vi "initialize_driver_session.vi"(4 "Supported instruments":string[](array[string]), 5 "Repeated Capabilities":T3(array[cluster]), 6 "Attributes":T1(array[cluster]) {"Access" items=["Read Only", "Write Only", "Read/Write"]; "Data Type" items=["ViInt32", "ViReal64", "ViString", "ViBoolean", "None"]}, 7 "Range Tables":T2(array[cluster]) {"Type" items=["Range", "Coerced", "Discrete"]}, 8 "error in":errorcluster, 9 "Option String":string, 11 "VISA resource name":refnum<visa-resource-name>) -> (0 "error out":errorcluster, 2 "Simulation *IDN? response":string, 3 "VISA resource name out":refnum<visa-resource-name>)   [LabVIEW 2014, in "rszvl_rsidr_core.lvlib"]
uses:
  rszvl_rsidr_core.lvlib
  type_Session_Data.ctl
  type_Error_Codes.ctl
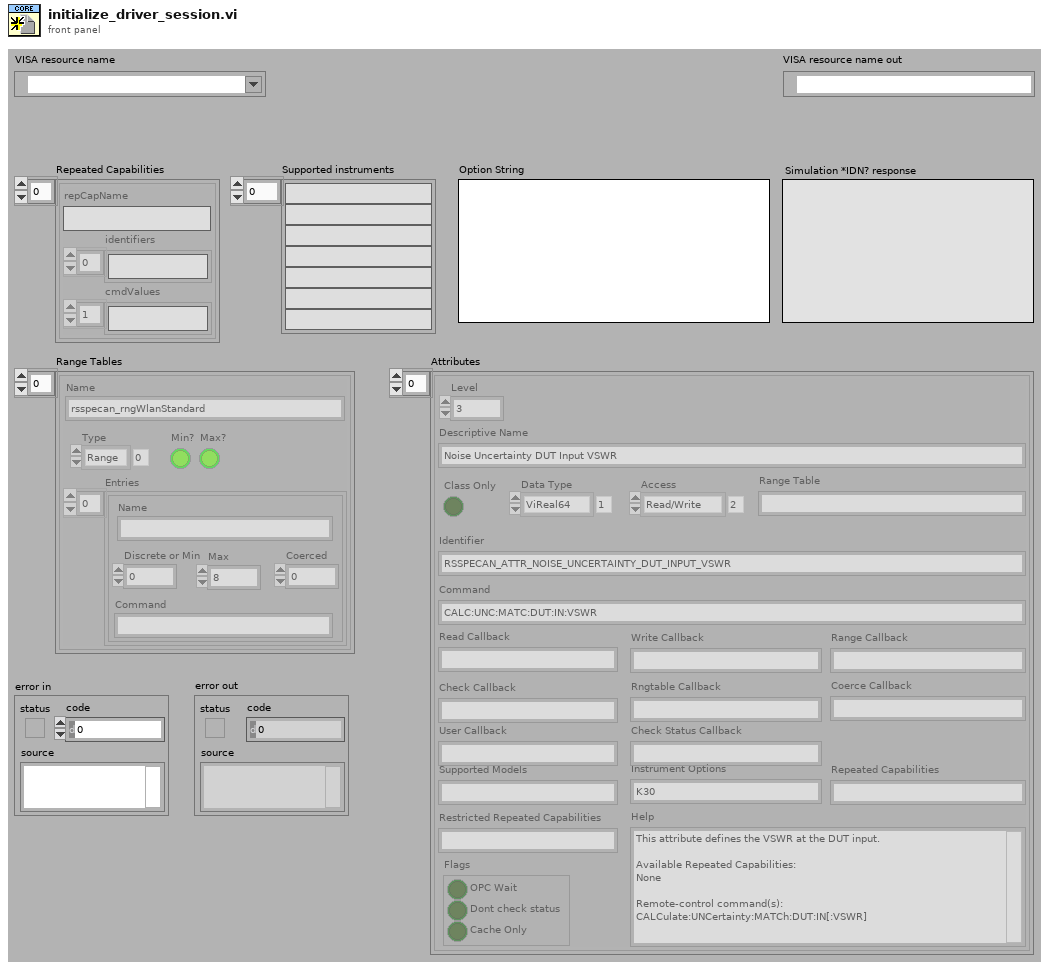
[diagram p1: front panel]
types:
  T1 = cluster{"Level":i32, "Descriptive Name":string, "Class Only":bool, "Data Type":u16, "Access":u16, "Identifier":string, "Range Table":string, "Command":string, "Read Callback":string, "Write Callback":string, "Range Callback":string, "Check Callback":string, "Rngtable Callback":string, "Coerce Callback":string, "User Callback":string, "Supported Models":string, "Instrument Options":string, "Repeated Capabilities":string, "Restricted Repeated Capabilities":string, "Help":string, "Flags":cluster{"OPC Wait":bool, "Dont check status":bool, "Cache Only":bool}, "Check Status Callback":string}[]
  T2 = cluster{"Name":string, "Type":i32, "Min?":bool, "Max?":bool, "Entries":cluster{"Name":string, "Discrete or Min":dbl, "Max":dbl, "Coerced":dbl, "Command":string}[]}[]
  T3 = cluster{"repCapName":string, "identifiers":string[], "cmdValues":string[]}[]
  T4 = typedef "rszvl_rsidr_core.lvlib/type_Error_Codes.ctl" = enum16{"No_error", "VISA_err_ResourceNotFound", "VISA_err_Timeout", "VISA_warn_MoreDataAvailable", "RS_err_MissingCallback", "RS_err_InvalidAttribute", "RS_err_InvalidValue", "RS_err_UnknownResource", "RS_err_AlreadyInitialized", "RS_err_InstrumentStatus", "RS_err_BadRepCapName", "RS_err_TypesMismatch", "RS_err_ValueNotSupported", "RS_err_InvalidRngTable", "RS_err_IDqueryFail", "RS_err_UnexpResponse", "VISA_warn_ConfigNotLoaded", "RS_err_AttributeNotReadable", "RS_err_AttributeNotWritable", "RS_err_InstrumentType", "RS_err_InstrumentOption", "VISA_err_InvalidSize", "RS_err_ReliabilityIndicator", "VISA_warn_UnknownStatus", "VISA_warn_TermCharRead", "VISA_err_IO_error"}
  T5 = enum16{"Initialize", "Check", "Get Numeric Value", "Get Default Value"}
  T6 = typedef "rszvl_rsidr_core.lvlib/type_Session_Data.ctl" = cluster{"Instr type":string, "Instr type for err. msg.":string, "Installed Options":string[], "OPC Timeout":i32, "Query Instrument Status":bool, "Check Range":bool, "Check Options":bool, "Add LF to Write":bool, "Simulate":bool, "Logging":bool, "Logging params":variant, "Interface Type":enum16{"Unknown", "GPIB", "VXI", "GPIB_VXI", "ASRL", "PXI", "TCPIP", "USB", "SOCKET"}, "Fast Sweep":i32, "AdditionalFlags":i32, "WaitBeforeWrite":i32, "WaitBeforeRead":i32, "BinDataChunkSize":i64}
  T7 = enum16{"Initialize", "GetData", "SetData", "Clear"}
  T8 = enum16{"Initialize", "Get Cached Value", "Set Cached Value", "Clear"}
  T9 = enum16{"Unknown", "GPIB", "VXI", "GPIB_VXI", "ASRL", "PXI", "TCPIP", "USB", "SOCKET"}
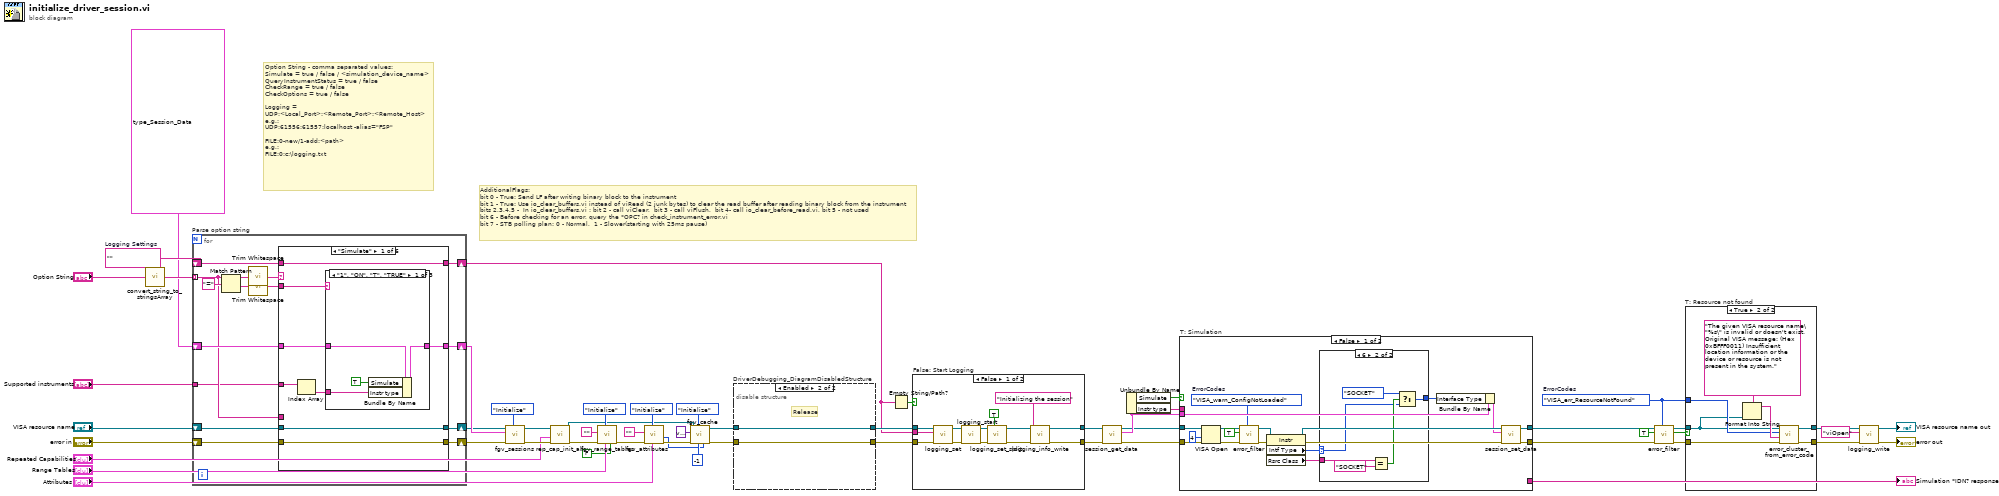
[diagram p0: block diagram]
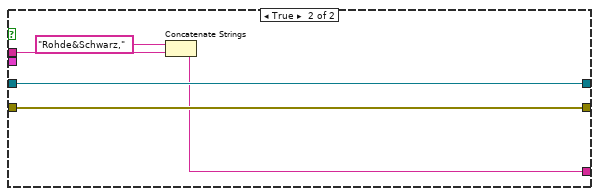
[diagram p3: hidden frame]
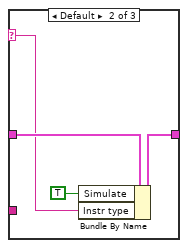
[diagram p6: hidden frame]
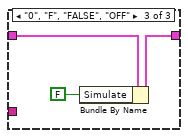
[diagram p7: hidden frame]
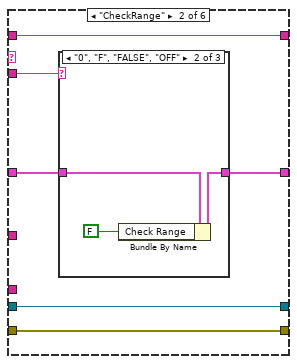
[diagram p8: hidden frame]
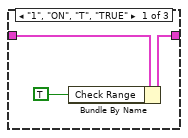
[diagram p9: hidden frame]
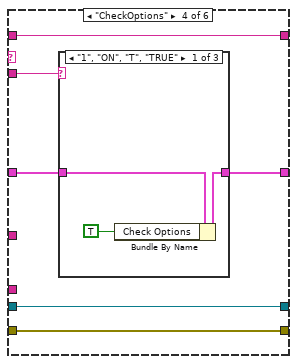
[diagram p12: hidden frame]
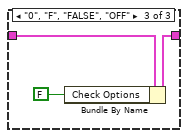
[diagram p14: hidden frame]
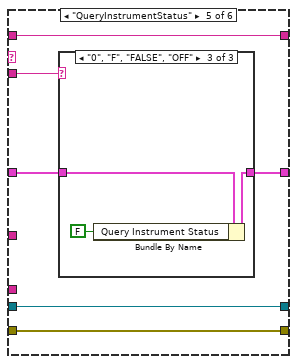
[diagram p15: hidden frame]
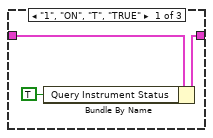
[diagram p16: hidden frame]
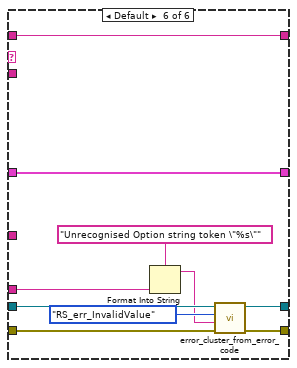
[diagram p18: hidden frame]
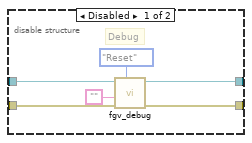
[diagram p19: hidden frame]
diagram:
  w17 = type_Error_Codes."VISA_err_ResourceNotFound"  # ErrorCodes
  w29 = ""  # Logging Settings
  # "AdditionalFlags:\nbit 0 - True: Send LF after writing binary block to the instrument\nbit 1 - True: Use io_clear_buffers.vi instead of viRead (2 junk bytes) to clear the read buffer after reading binary block from the instrument\nbits 2,3,4,5 -  In io_clear_buffers.vi : bit 2 - call viClear,  bit 3 - call viFlush,  bit 4- call io_clear_before_read.vi, bit 5 - not used\nbit 6 - Before checking for an error, query the *OPC? in check_instrument_error.vi\nbit 7 - STB polling plan: 0 - Normal,  1 - Slower(starting with 25ms pause)"
  # "Option String - comma separated values:\nSimulate = true / false / <simulation_device_name>\nQueryInstrumentStatus = true / false\nCheckRange = true / false\nCheckOptions = true / false\n\nLogging =\nUDP:<Local_Port>:<Remote_Port>:<Remote_Host>\ne.g.:\nUDP:61556:61557:localhost -alias=\"FSP\"\n\nFILE:0-new/1-add:<path>\ne.g.:\nFILE:0:c:\\logging.txt"
  n1 = call "convert_string_to_stringsArray.vi"("String in"="Option String") -> ("string array out"=w38:string[])  [unwired: 3 in, 1 out]
  n2 = for "Parse option string" {
    tunnel: w38 -> [w60] mode=indexing
    shift-right: [w66] -> w37
    shift-left: T6 {"Instr type"="", "Instr type for err. msg."="", "Installed Options"=[], "OPC Timeout"=5000, "Query Instrument Status"=TRUE, "Check Range"=TRUE, "Check Options"=TRUE, "Add LF to Write"=FALSE, "Simulate"=FALSE, "Logging"=FALSE, "Logging params"=variant, "Interface Type"=enum."TCPIP", "Fast Sweep"=0, "AdditionalFlags"=4, "WaitBeforeWrite"=0, "WaitBeforeRead"=0, "BinDataChunkSize"=10000000} ("Session User Data in") -> [w67]
    shift-right: [w63] -> w33
    shift-left: "error in" -> [w64]
    shift-right: [w61] -> w34
    shift-left: "VISA resource name" -> [w62]
    tunnel: "Supported instruments" -> [w58]
    shift-right: [w56] -> w27
    shift-left: w29 -> [w57]
    n3 = Match Pattern(string=w60, regular expression="=") -> (before substring=w69:string, after substring=w68:string)  [unwired: 1 in, 2 out]
    n4 = call "Trim Whitespace.vi"("string"=w69) -> ("trimmed string"=w65:string)  [unwired: 1 in]
    n5 = call "Trim Whitespace.vi"("string"=w68) -> ("trimmed string"=w59:string)  [unwired: 1 in]
    n6 = case shown="\"Simulate\"" w65 {
      tunnel: w67 -> [w78 w95 w103 w112 w125 w134]
      tunnel: [w77 w94 w103 w111 w124 w134] -> w66
      tunnel: w64 -> [w73 w92 w106 w109 w122 w141]
      tunnel: [w73 w92 w106 w109 w122 w140] -> w63
      tunnel: w62 -> [w72 w91 w105 w108 w121 w139]
      tunnel: [w72 w91 w105 w108 w121 w138] -> w61
      tunnel: w60 -> [_ _ _ _ _ w136]
      tunnel: w59 -> [w74 w93 w104 w110 w123 _]
      tunnel: w58 -> [w76 _ _ _ _ _]
      tunnel: w57 -> [w71 w90 _ w107 w120 w133]
      tunnel: [w71 w90 w104 w107 w120 w133] -> w56
      frame "Simulate" {
        n7 = Index Array(array=w76) -> (element=w75:string)  [unwired: 1 in]
        n8 = case shown="\"1\", \"ON\", \"T\", \"TRUE\"" w74 {
          selector: w74 -> [_ w83 _]
          tunnel: w78 -> [w82 w86 w89]
          tunnel: [w81 w85 w88] -> w77
          tunnel: w75 -> [w80 _ _]
          frame "1", "ON", "T", "TRUE" {
            n9 = Bundle By Name(cluster=w82, "Simulate"=TRUE ("Simulation"), "Instr type"=w80) -> (w81:T6)
          }
          frame Default {
            n10 = Bundle By Name(cluster=w86, "Simulate"=TRUE ("Simulation"), "Instr type"=w83) -> (w85:T6)
          }
          frame "0", "F", "FALSE", "OFF" {
            n11 = Bundle By Name(cluster=w89, "Simulate"=FALSE ("Simulation")) -> (w88:T6)
          }
        }
      }
      frame "CheckRange" {
        n12 = case shown="\"0\", \"F\", \"FALSE\", \"OFF\"" w93 {
          tunnel: w95 -> [w98 w101 w102]
          tunnel: [w97 w100 w102] -> w94
          frame "1", "ON", "T", "TRUE" {
            n13 = Bundle By Name(cluster=w98, "Check Range"=TRUE ("Simulation")) -> (w97:T6)
          }
          frame "0", "F", "FALSE", "OFF" {
            n14 = Bundle By Name(cluster=w101, "Check Range"=FALSE ("Simulation")) -> (w100:T6)
          }
          frame Default {
          }
        }
      }
      frame "Logging" {
      }
      frame "CheckOptions" {
        n15 = case shown="\"1\", \"ON\", \"T\", \"TRUE\"" w110 {
          tunnel: w112 -> [w115 w116 w119]
          tunnel: [w114 w116 w118] -> w111
          frame "1", "ON", "T", "TRUE" {
            n16 = Bundle By Name(cluster=w115, "Check Options"=TRUE ("Simulation")) -> (w114:T6)
          }
          frame Default {
          }
          frame "0", "F", "FALSE", "OFF" {
            n17 = Bundle By Name(cluster=w119, "Check Options"=FALSE ("Simulation")) -> (w118:T6)
          }
        }
      }
      frame "QueryInstrumentStatus" {
        n18 = case shown="\"0\", \"F\", \"FALSE\", \"OFF\"" w123 {
          tunnel: w125 -> [w128 w129 w132]
          tunnel: [w127 w129 w131] -> w124
          frame "1", "ON", "T", "TRUE" {
            n19 = Bundle By Name(cluster=w128, "Query Instrument Status"=TRUE ("Simulation")) -> (w127:T6)
          }
          frame Default {
          }
          frame "0", "F", "FALSE", "OFF" {
            n20 = Bundle By Name(cluster=w132, "Query Instrument Status"=FALSE ("Simulation")) -> (w131:T6)
          }
        }
      }
      frame Default {
        n21 = Format Into String(format string="Unrecognised Option string token \"%s\"", w136) -> (resulting string=w135:string)  [unwired: 2 in, 1 out]
        n22 = call "error_cluster_from_error_code.vi"("error in"=w141, "error message (\"\")"=w135, "Error Enum in"=type_Error_Codes."RS_err_InvalidValue", "VISA resource name"=w139) -> ("error out"=w140:errorcluster, "VISA resource name out"=w138:refnum<visa-resource-name>)  [unwired: 6 in]
      }
    }
  }
  n23 = call "fgv_sessions.vi"("Operation"=T7."Initialize", "error in"=w33, "Session User Data in (None)"=w37, "VISA resource name"=w34) -> ("error out"=w25:errorcluster, "VISA resource name out"=w24:refnum<visa-resource-name>)  [unwired: 5 in, 1 out]
  n24 = call "rep_cap_init_all.vi"("error in"=w25, "Repeated Capabilities"="Repeated Capabilities", "VISA resource name"=w24) -> ("error out"=w26:errorcluster, "VISA resource name out"=w23:refnum<visa-resource-name>)  [unwired: 7 in]
  n25 = call "fgv_range_tables.vi"("Range Checking"=FALSE ("Range Checking Disabled"), "Range Tables (Empty)"="Range Tables", "Operation"=T5."Initialize", "error in"=w26, "Range Table ID in"="" ("Empty String Constant")) -> ("error out"=w50:errorcluster)  [unwired: 3 in, 3 out]
  n26 = call "fgv_attributes.vi"("Attributes (Empty)"="Attributes", "Operation"=enum16{"Initialize", "Get Attribute"}."Initialize", "error in"=w50, "Attribute ID in"="" ("Empty String Constant")) -> ("error out"=w49:errorcluster, "Count out"=w48:i32)  [unwired: 5 in, 1 out]
  n27 = call "fgv_cache.vi"("Initialization Count (0)"=w48, "Index in"=-1, "Operation"=T8."Initialize", "error in"=w49, "Value in"=variant, "VISA resource name"=w23) -> ("error out"=w41:errorcluster, "VISA resource name out"=w40:refnum<visa-resource-name>)  [unwired: 3 in, 1 out]
  n28 = disable-structure "DriverDebugging_DiagramDisabledStructure" shown="Enabled" {
    disable-tunnel: w41 -> [w147 w149]
    disable-tunnel: [w145 w149] -> w31
    disable-tunnel: w40 -> [w146 w150]
    disable-tunnel: [w144 w150] -> w30
    frame Disabled {
      # "Debug"
      n29 = call "fgv_debug.vi"("Operation"=enum16{"Reset", "ReadCommand", "SetCommand"}."Reset", "error in"=w147, "Command in"="" ("Empty String Constant"), "VISA resource name"=w146) -> ("error out"=w145:errorcluster, "VISA resource name out"=w144:refnum<visa-resource-name>)  [unwired: 6 in]
    }
    frame Enabled {
      # "Release"
    }
  }
  n30 = Empty String/Path?(string/path=w27) -> (empty?=w28:bool)
  n31 = case "False: Start Logging" shown="False" w28 {
    tunnel: w31 -> [w161 w164]
    tunnel: w30 -> [w160 w165]
    tunnel: [w153 w164] -> w15
    tunnel: [w152 w165] -> w14
    tunnel: w27 -> [w163 _]
    frame False {
      n32 = call "logging_set.vi"("error in"=w161, "Logging target"=w163, "VISA resource name"=w160) -> ("error out"=w159:errorcluster, "VISA resource name out"=w158:refnum<visa-resource-name>)  [unwired: 7 in]
      n33 = call "logging_start.vi"("error in"=w159, "VISA resource name"=w158) -> ("error out"=w157:errorcluster, "VISA resource name out"=w156:refnum<visa-resource-name>)  [unwired: 8 in]
      n34 = call "logging_set_split.vi"("Evaluate section error (F)"=TRUE, "error in"=w157, "VISA resource name"=w156) -> ("error out"=w155:errorcluster, "VISA resource name out"=w154:refnum<visa-resource-name>)  [unwired: 7 in]
      n35 = call "logging_info_write.vi"("error in"=w155, "String to write"="Initializing the session", "VISA resource name"=w154) -> ("error out"=w153:errorcluster, "VISA resource name out"=w152:refnum<visa-resource-name>)  [unwired: 7 in]
    }
    frame True {
    }
  }
  n36 = call "session_get_data.vi"("error in"=w15, "VISA resource name"=w14) -> ("error out"=w13:errorcluster, "Session User Data out"=w16:T6, "VISA resource name out"=w12:refnum<visa-resource-name>)  [unwired: 7 in]
  n37 = Unbundle By Name(w16) -> ("Simulate"=w11:bool, "Instr type"=w18:string)
  n38 = case "T: Simulation" shown="False" w11 {
    tunnel: w12 -> [w181 w194]
    tunnel: w13 -> [w182 w195]
    tunnel: [w173 w195] -> w10
    tunnel: [w172 w194] -> w3
    tunnel: w18 -> [_ w192]
    tunnel: [_ w191] -> w9
    tunnel: w16 -> [w176 _]
    frame False {
      w171 = type_Error_Codes."VISA_warn_ConfigNotLoaded"  # ErrorCodes
      n39 = VISA Open ("Open instrument")(access mode=u32 4, error in (no error)=w182, VISA resource name=w181) -> (VISA resource name=w169:refnum<visa-resource-name>, error out=w170:errorcluster)  [unwired: 2 in]
      n40 = call "error_filter.vi"("Error Enum in"=w171, "error in"=w170, "Clear detected code (F)"=TRUE, "VISA resource name"=w169) -> ("error out"=w168:errorcluster, "VISA resource name out"=w167:refnum<visa-resource-name>)  [unwired: 5 in, 1 out]
      n41 = property on="Property Node" class="Instr"(reference=w167, error in=w168) -> (reference out=w179:refnum<visa-resource-name>, error out=w180:errorcluster, "Intf Type"=w178:u16, "Rsrc Class"=w177:string)
      n42 = case shown="6" w178 {
        selector: w178 -> [w184 w187]
        tunnel: w177 -> [_ w190]
        tunnel: [w184 w186] -> w174
        frame Default {
        }
        frame 6 {
          n43 = Equal?(x=w190, y="SOCKET") -> (x = y?=w188:bool)
          n44 = Select(t=T9."SOCKET" ("Interface Type"), s=w188, f=w187) -> (s? t:f=w186:u16)
        }
      }
      n45 = Bundle By Name(cluster=w176, "Interface Type"=w174) -> (w175:T6)
      n46 = call "session_set_data.vi"("error in"=w180, "Session User Data in"=w175, "VISA resource name"=w179) -> ("error out"=w173:errorcluster, "VISA resource name out"=w172:refnum<visa-resource-name>)  [unwired: 7 in]
    }
    frame True {
      n47 = Concatenate Strings("Rohde&Schwarz," ("read buffer"), w192) -> (w191:string)
    }
  }
  "Simulation *IDN? response" <- w9
  n48 = call "error_filter.vi"("Error Enum in"=w17, "error in"=w10, "Clear detected code (F)"=TRUE, "VISA resource name"=w3) -> ("error out"=w20:errorcluster, "Code Detected"=w21:bool, "VISA resource name out"=w2:refnum<visa-resource-name>)  [unwired: 5 in]
  n49 = case "T: Resource not found" shown="True" w21 {
    tunnel: w20 -> [w197 w202]
    tunnel: [w197 w204] -> w7
    tunnel: w2 -> [w196 w198]
    tunnel: w17 -> [_ w200]
    tunnel: [w196 w199] -> w6
    frame False {
    }
    frame True {
      n50 = Format Into String(format string="The given VISA resource name\"%s\" is invalid or doesn't exist. Original VISA message: (Hex 0xBFFF0011) Insufficient location information or the device or resource is not present in the system.", w198) -> (resulting string=w201:string)  [unwired: 2 in, 1 out]
      n51 = call "error_cluster_from_error_code.vi"("error in"=w202, "error message (\"\")"=w201, "Error Enum in"=w200, "VISA resource name"=w198) -> ("error out"=w204:errorcluster, "VISA resource name out"=w199:refnum<visa-resource-name>)  [unwired: 6 in]
    }
  }
  n52 = call "logging_write.vi"("error in"=w7, "String to write"="viOpen", "VISA resource name"=w6) -> ("error out"=→"error out":errorcluster, "VISA resource name out"=→"VISA resource name out":refnum<visa-resource-name>)  [unwired: 7 in]
